vi "Intsy_updateChanStream.vi"(8 "error in (no error)":errorcluster, 10 "ChanSelString":string, 11 "VISA resource name":refnum<visa-resource-name>) -> (0 "error out":errorcluster, 2 "NChansInStream":i32, 3 "VISA resource name out":refnum<visa-resource-name>, 4 "NStreamChansString":string)   [LabVIEW 2020]
doc: "Trigger streaming channels update to Teensy. Upon request, the Teensy Tx buffer is first flushed. Then we process responses from Teensy to enter 5x uint32 elements, in comma separated string. Each of these uint32 are bitmasks for amps A-D (first 4) and the last is for accelx,y,z and Vdd. Lastly teensy responds with the number of channels it will stream, which may be less than requested if the user asked for more than the max possible at this streaming rate.\n\nNOTE: this VI enabled VISA reads to terminate with Termination Character of 0x04. For resuming VISA reads for data streaming, the termination character must be DISABLED. Set properties TermChar En = False; ASRL End In = none."
uses:
  <vilib>/Instr/_visa.llb/VISA Flush IO Buffer Mask.ctl
panel:
  out "iter":i32
  out "enterMatchIndex":i32
  out "BytesAtPortBeforeFlush":u32
  out "x bytes written":u32
  out "Nchansreply":string
  out "setchansReqReply":string
  in  "updateStreamChansChar":string="h"
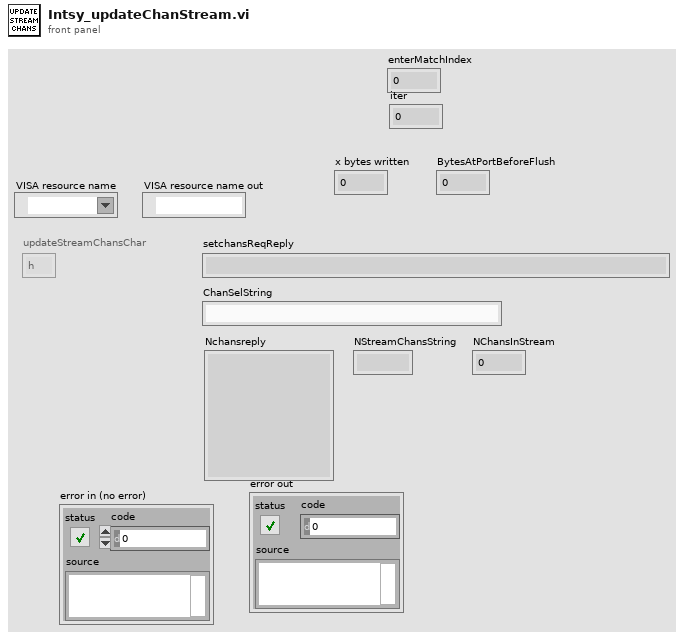
[diagram p1: front panel]
types:
  T1 = typedef "VISA Flush IO Buffer Mask.ctl" = u16
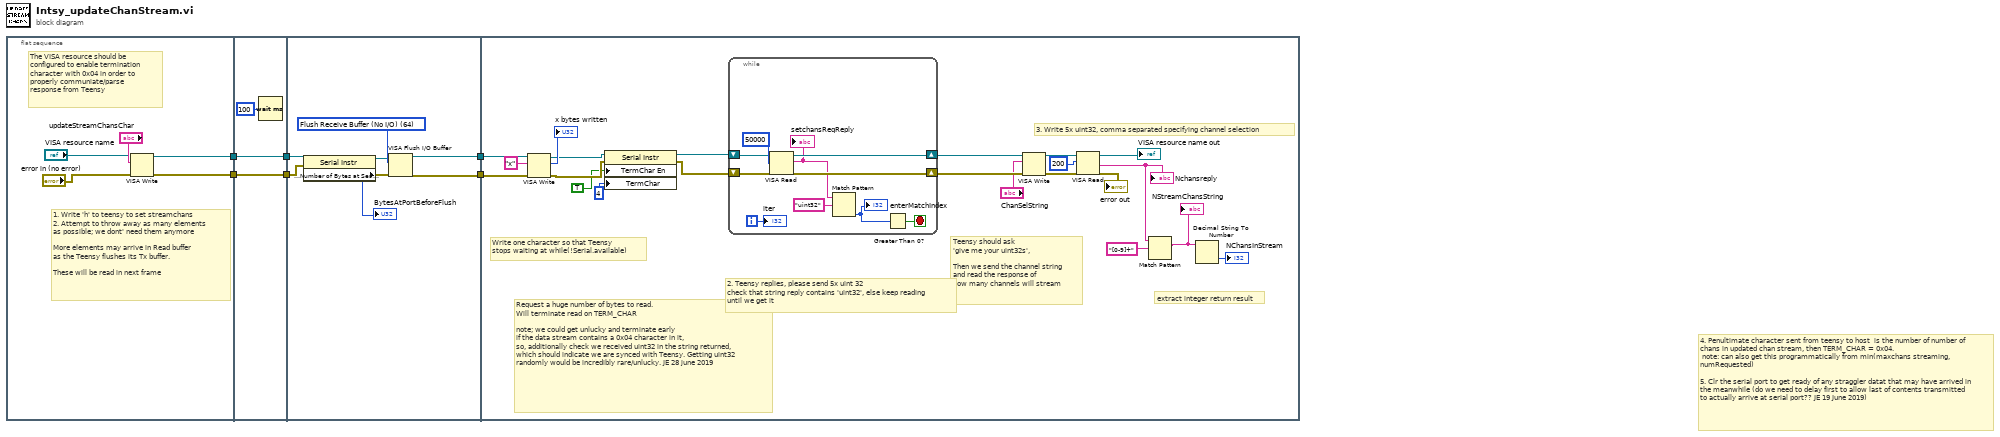
[diagram p0: block diagram]
diagram:
  # "4. Penultimate character sent from teensy to host  is the number of number of chans in updated chan stream, then TERM_CHAR = 0x04.\n note: can also get this programmatically from min(maxchans streaming, numRequested) \n\n5. Clr the serial port to get ready of any straggler datat that may have arrived in the meanwhile (do we need to delay first to allow last of contents transmitted to actually arrive at serial port?? JE 19 June 2019)"
  n1 = flat-sequence {
    tunnel: [w8] -> w5
    tunnel: [w7] -> w3
    tunnel: [w13] -> w6
    tunnel: w5 -> [w13]
    tunnel: [w12] -> w4
    tunnel: w3 -> [w12]
    tunnel: w6 -> [w18]
    tunnel: w4 -> [w21]
    tunnel: [w16] -> w2
    tunnel: [w15] -> w1
    tunnel: w2 -> [w25]
    tunnel: w1 -> [w24]
    frame #0 {
      # "The VISA resource should be configured to enable termination character with 0x04 in order to properly communiate/parse response from Teensy"
      # "1. Write 'h' to teensy to set streamchans\n2. Attempt to throw away as many elements \nas possible; we dont' need them anymore\n\nMore elements may arrive in Read buffer\nas the Teensy flushes its Tx buffer.\n\nThese will be read in next frame"
      n2 = VISA Write(VISA resource name="VISA resource name", write buffer="updateStreamChansChar", error in (no error)="error in (no error)") -> (VISA resource name out=w7:refnum<visa-resource-name>, error out=w8:errorcluster)  [unwired: 1 out]
    }
    frame #1 {
      n3 = Wait (ms)(milliseconds to wait=u32 100) -> ()  [unwired: 1 out]
    }
    frame #2 {
      w22 = T1 64 items=["Flush Receive Buffer"=16, "Write Transmit Buffer to Device"=32, "Flush Receive Buffer (No I/O)"=64, "Flush Transmit Buffer"=128] ("Mask")
      n4 = property class="Serial Instr"(reference=w21, error in=w18) -> (reference out=w20:refnum<visa-resource-name>, error out=w19:errorcluster, "Serial Settings:Number of Bytes at Serial Port"=→"BytesAtPortBeforeFlush":u32)
      n5 = VISA Flush I/O Buffer(VISA resource name=w20, mask (16)=w22, error in (no error)=w19) -> (VISA resource name out=w16:refnum<visa-resource-name>, error out=w15:errorcluster)
    }
    frame #3 {
      # "2. Teensy replies, please send 5x uint 32\ncheck that string reply contains 'uint32', else keep reading\nuntil we get it"
      # "Write one character so that Teensy\nstops waiting at while(!Serial.available)"
      # "Request a huge number of bytes to read.\nWill terminate read on TERM_CHAR\n\nnote; we could get unlucky and terminate early\nif the data stream contains a 0x04 character in it,\nso, additionally check we received uint32 in the string returned,\nwhich should indicate we are synced with Teensy. Getting uint32\nrandomly would be incredibly rare/unlucky. JE 28 june 2019"
      # "Teensy should ask\n'give me your uint32s',\n\nThen we send the channel string\nand read the response of \nhow many channels will stream"
      # "extract integer return result"
      # "3. Write 5x uint32, comma separated specifying channel selection"
      n6 = VISA Write(VISA resource name=w25, write buffer="x", error in (no error)=w24) -> (VISA resource name out=w29:refnum<visa-resource-name>, return count=→"x bytes written":u32, error out=w28:errorcluster)
      n7 = property class="Serial Instr"(reference=w29, error in=w28, "TermChar En"=TRUE ("Message Based Settings:Termination Character Enable"), "TermChar"=u8 4 ("Message Based Settings:Termination Character")) -> (reference out=w31:refnum<visa-resource-name>, error out=w30:errorcluster)
      n8 = while {
        shift-right: [w52] -> w32
        shift-left: w31 -> [w50]
        shift-right: [w54] -> w42
        shift-left: w30 -> [w49]
        i -> [w45]
        stop <- w46 stop-if-true
        n9 = VISA Read(VISA resource name=w50, byte count=u32 50000, error in (no error)=w49) -> (VISA resource name out=w52:refnum<visa-resource-name>, read buffer=w48:string, error out=w54:errorcluster)  [unwired: 1 out]
        "setchansReqReply" <- w48
        n10 = Match Pattern(string=w48, regular expression="uint32") -> (offset past match=w47:i32)  [unwired: 1 in, 3 out]
        "enterMatchIndex" <- w47
        n11 = Greater Than 0?(x=w47) -> (x > 0?=w46:bool)
        "iter" <- w45
      }
      n12 = VISA Write(VISA resource name=w32, write buffer="ChanSelString", error in (no error)=w42) -> (VISA resource name out=w37:refnum<visa-resource-name>, error out=w38:errorcluster)  [unwired: 1 out]
      n13 = VISA Read(VISA resource name=w37, byte count=u32 200, error in (no error)=w38) -> (VISA resource name out=→"VISA resource name out":refnum<visa-resource-name>, read buffer=w43:string, error out=→"error out":errorcluster)  [unwired: 1 out]
      "Nchansreply" <- w43
      n14 = Match Pattern(string=w43, regular expression="[0-9]+") -> (match substring=w44:string)  [unwired: 1 in, 3 out]
      "NStreamChansString" <- w44
      n15 = Decimal String To Number(string=w44) -> (number=→"NChansInStream":i32)  [unwired: 2 in, 1 out]
    }
  }
